vi "PC to cDAQ fglbl.vi"(5 "message":T3, 7 "cDAQ Thread":T4, 8 "error in (no error)":errorcluster, 10 "tcp connection info":T1) -> (0 "error out":errorcluster)   [LabVIEW 2012]
uses:
  interthread comms/typedefs/state queue fglbl actions.ctl
  interthread comms/typedefs/interthread message.ctl
  typedefs/connection type.ctl
  typedefs/tcp connection info.ctl
  interthread comms/typedefs/app type.ctl
  typedefs/interapp tx message request.ctl
  interthread comms/typedefs/HMI PC thread IDs.ctl
  interthread comms/typedefs/station cDAQ thread IDs.ctl
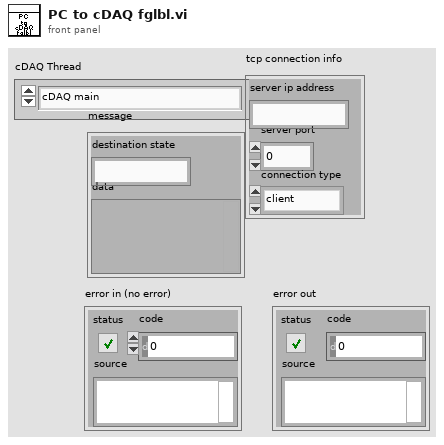
[diagram p1: front panel]
types:
  T1 = typedef "tcp connection info.ctl" = cluster{"server ip address":string, "server port":i32, "connection type":T2}
  T2 = typedef "connection type.ctl" = enum16{"client", "server"}
  T3 = typedef "interthread message.ctl" = cluster{"destination state":string, "data":variant}
  T4 = typedef "station cDAQ thread IDs.ctl" = enum16{"cDAQ main", "analog input", "eol test exe", "nvh test exe", "tcp comms"}
  T5 = typedef "app type.ctl" = enum16{"PC", "cDAQ", "AuditHMI"}
  T6 = typedef "interapp tx message request.ctl" = cluster{"destination app":T5, "destination thread":string, "tcp connection info":T1, "message":T3}
  T7 = typedef "state queue fglbl actions.ctl" = enum16{"init queues", "get queue ref", "destroy queues"}
  T8 = typedef "HMI PC thread IDs.ctl" = enum16{"hmi main", "file output", "tcp comms", "NVH process"}
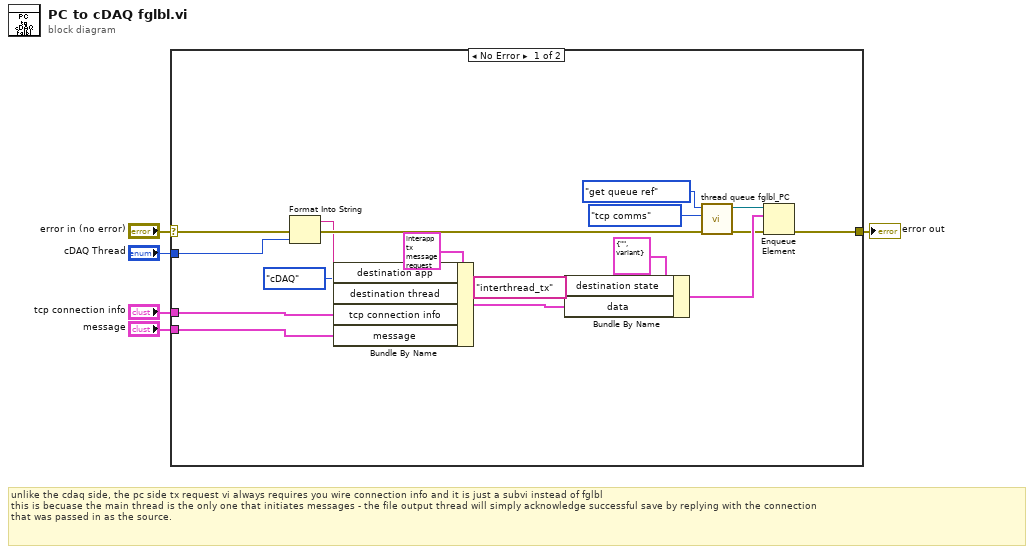
[diagram p0: block diagram]
diagram:
  # "unlike the cdaq side, the pc side tx request vi always requires you wire connection info and it is just a subvi instead of fglbl\nthis is becuase the main thread is the only one that initiates messages - the file output thread will simply acknowledge successful save by replying with the connection\nthat was passed in as the source."
  n1 = case shown="No Error" "error in (no error)" {
    selector: "error in (no error)" -> [w19 w23]
    tunnel: [w22 w23] -> w5
    tunnel: "cDAQ Thread" -> [w21 _]
    tunnel: "message" -> [w20 _]
    tunnel: "tcp connection info" -> [w18 _]
    frame No Error {
      n2 = Format Into String(error in=w19, w21) -> (resulting string=w16:string, error out=w17:errorcluster)  [unwired: 2 in]
      n3 = Bundle By Name(cluster=T6 {"destination app"=enum."PC", "destination thread"="", "tcp connection info"={"server ip address"="", "server port"=0, "connection type"=enum."client"}, "message"={"destination state"="", "data"=variant}}, "destination app"=app_type."cDAQ", "destination thread"=w16, "tcp connection info"=w18, "message"=w20) -> (w14:T6)
      n4 = Bundle By Name(cluster=T3 {"destination state"="", "data"=variant} ("message"), "destination state"="interthread_tx", "data"=w14) -> (w12:T3)
      n5 = call "thread queue fglbl_PC.vi"("error in (no error)"=w17, "Station cDAQ Thread Queue"=HMI_PC_thread_IDs."tcp comms", "action"=state_queue_fglbl_actions."get queue ref") -> ("error out"=w8:errorcluster, "queue out"=w9:refnum<queue>)  [unwired: 6 in, 1 out]
      n6 = Enqueue Element(queue=w9, element=w12, error in (no error)=w8) -> (error out=w22:errorcluster)  [unwired: 1 in, 2 out]
    }
    frame Error {
    }
  }
  "error out" <- w5
